vi "Clean and Run Build Spec.vi"(8 "error in (no error)":errorcluster, 9 "Target":T1, 10 "Name of build specification":string, 11 "Path to project":path) -> (0 "error out":errorcluster, 2 "Generated files":path[](array[path]))   [LabVIEW 2017]
uses:
  Target Type.ctl
  Constants.vi
  <vilib>/AppBuilder/AB_API_Simple/Build (path).vi
  <vilib>/AppBuilder/AB_API_Simple/NI_App_Builder_API.lvlib
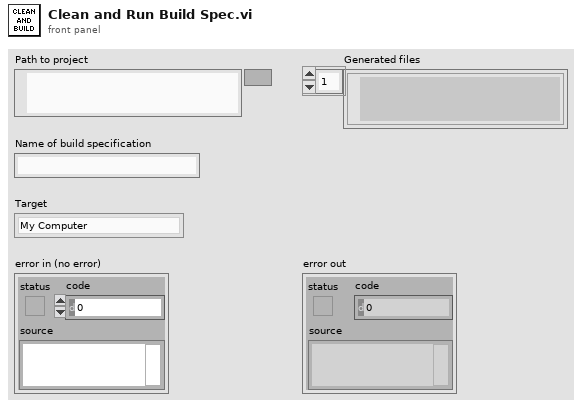
[diagram p1: front panel]
types:
  T1 = typedef "Target Type.ctl" = enum16{"My Computer", "Pharlap"}
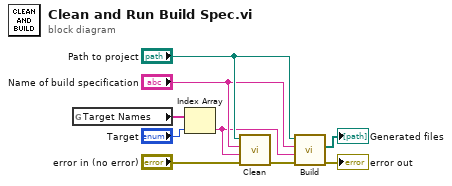
[diagram p0: block diagram]
diagram:
  n1 = global read "Constants.vi" "Target Names"() -> (w1:string[])
  n2 = Index Array(array=w1, index="Target") -> (element=w3:string)
  n3 = call <vilib>:"Clean.vi"("error in (no error)"="error in (no error)", "Name of target (My Computer)"=w3, "Name of build specification (if empty: clean all)"="Name of build specification", "Path to project"="Path to project") -> ("error out"=w9:errorcluster)  [unwired: 7 in]
  n4 = call-poly <vilib>:"Build.vi"("error in (no error)"=w9, "Name of target (My Computer)"=w3, "Name of build specification (if empty: build all)"="Name of build specification", "Path to project"="Path to project") -> ("error out"=→"error out":errorcluster, "Generated files"=→"Generated files":path[])  [unwired: 6 in]
